vi "MakeImageFreqArray.vi"(11 "Top Sponsor Image List":T1) -> (3 "Cluster":cluster{T2[], "Frequency (s)":dbl})   [LabVIEW 2013]
uses:
  <vilib>/picture/picture.llb/imagedata.ctl
  ImageInfoList.ctl
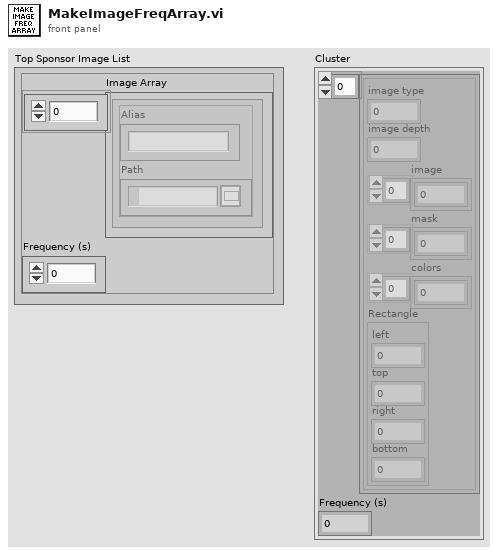
[diagram p1: front panel]
types:
  T1 = typedef "ImageInfoList.ctl" = cluster{"Image Array":cluster{"Alias":string, "Path":path}[], "Frequency (s)":dbl}
  T2 = typedef "imagedata.ctl" = cluster{"image type":i32, "image depth":i32, "image":u8[], "mask":u8[], "colors":u32[], "Rectangle":cluster{"left":i16, "top":i16, "right":i16, "bottom":i16}}
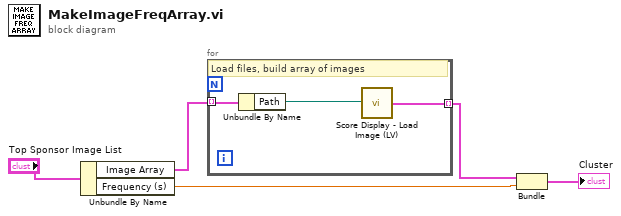
[diagram p0: block diagram]
diagram:
  n1 = Unbundle By Name("Top Sponsor Image List") -> ("Image Array"=w2:cluster{"Alias":string, "Path":path}[], "Frequency (s)"=w4:dbl)
  n2 = for {
    tunnel: [w8] -> w3 mode=indexing
    tunnel: w2 -> [w7] mode=indexing
    # "Load files, build array of images"
    n3 = Unbundle By Name(w7) -> ("Path"=w6:path)
    n4 = call "Score Display - Load Image (LV).vi"("path to image file"=w6) -> ("image data"=w8:T2)
  }
  n5 = Bundle(w3, "Frequency (s)"=w4) -> (→"Cluster":cluster{T2[], "Frequency (s)":dbl})  [unwired: 1 in]
